vi "lab1_usrp_byte_packet_transceiver.vi"() -> ()   [LabVIEW 2014]
uses:
  <vilib>/addons/Modulation/Analog/support/mod_Set Error Source.vi
  sub_var_stop.vi
  <vilib>/addons/Modulation/Digital/General/MT Generate PSK System Parameters(M).vi
  <vilib>/addons/Modulation/Digital/Support/Common/Validators/mod_Generate Filter Coefficients Validate.vi
  <vilib>/addons/Modulation/Digital/General/subVIs/mod_Generate Filter Coefficients.vi
  <vilib>/addons/Modulation/Digital/General/MT Apply Matched Filter (Generic).vi
  <vilib>/addons/Modulation/Digital/General/MT Align to Ideal Symbols (Generic).vi
  <vilib>/addons/Modulation/Digital/General/MT Map PSK Symbols to Bits.vi
  <instrlib>/niUSRP/niUSRP Fetch Rx Data (CDB Cluster).vi
  <instrlib>/niUSRP/niUSRP Write Tx Data (CDB Cluster).vi
  <vilib>/addons/Modulation/Digital/General/MT Map Bits to PSK Symbols.vi
  <vilib>/addons/Modulation/Digital/General/MT Apply Pulse Shaping Filter (Generic).vi
  <vilib>/addons/Modulation/niDMT.lvlib
panel:
  out "Received symbols":cdb[](graph)
  in  "Transmit power (db)":dbl
  out "History":string
  out "Constellation Map":cdb[](graph)
  out "Received texts":string
  out "Instant rx texts":string
  in  "Instant transmit message":string
  out "size(s) 4":i32
  in  "Send":bool
  out "# elements in buffer":i32
  in  "filter length (symbols)":i32=8
  in  "filter parameter":dbl=0.35 format="%.2f"
  in  "pulse shaping filter (none)":T1(ring)=enum."Raised Cosine"
  in  "M-PSK (4)":i32=4
  in  "samples per symbol (16)":i32=4
  in  "number of samples":i64=40000
  out "coerced gain 2":dbl format="%#_6f"
  out "coerced carrier frequency 2":dbl=915000000.0 format="%#_6p"
  out "coerced IQ rate 2":dbl=4000000.0 format="%#_6p"
  in  "active antenna 2":string="RX2"
  in  "gain 2":dbl format="%#_6f"
  in  "RX device names":refnum<k15>="192.168.10.2"
  out "coerced gain":dbl format="%#_6f"
  out "coerced carrier frequency":dbl=915000000.0 format="%#_6p"
  out "coerced IQ rate":dbl=4000000.0 format="%#_6p"
  in  "TX device names":refnum<k15>="192.168.10.2"
  in  "gain":dbl format="%#_6f"
  in  "carrier frequency":dbl=915000000.0 format="%#_6p"
  in  "IQ rate":dbl=1000000.0 format="%#_6p"
  in  "active antenna":string="TX1"
  in  "stop":bool
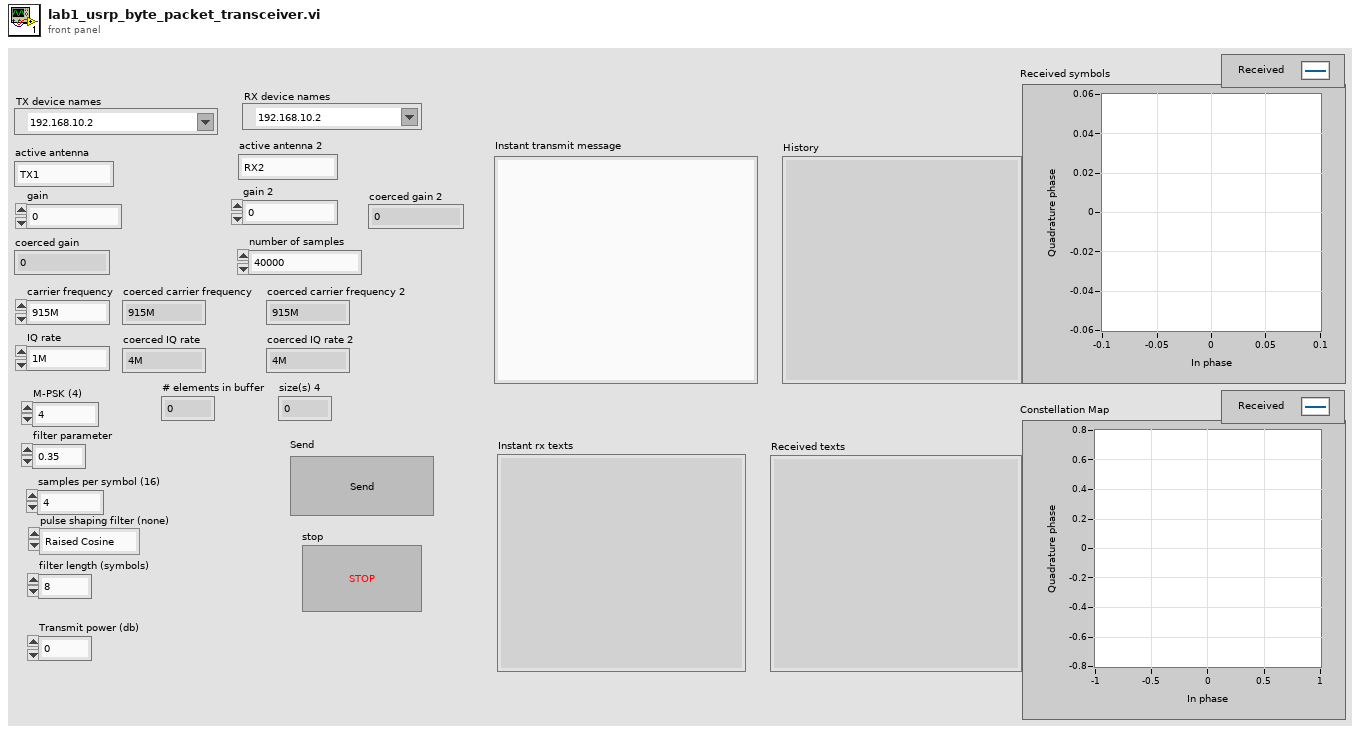
[diagram p1: front panel]
types:
  T1 = enum16{"none", "Raised Cosine", "Root Raised Cos", "Gaussian"}
  T2 = enum16{"FSK", "PSK", "QAM", "MSK", "PAM", "ASK", "CPM"}
  T3 = cluster{"samples per symbol (16)":i32, "symbol map":cdb[], "differential PSK":enum16{"disable", "enable"}, "PSK type":u16}
  T4 = typedef "niAMT.lvlib/Complex Data Waveform.ctl" = cluster{"t0":dbl, "dt":dbl, "Y":cdb[]}
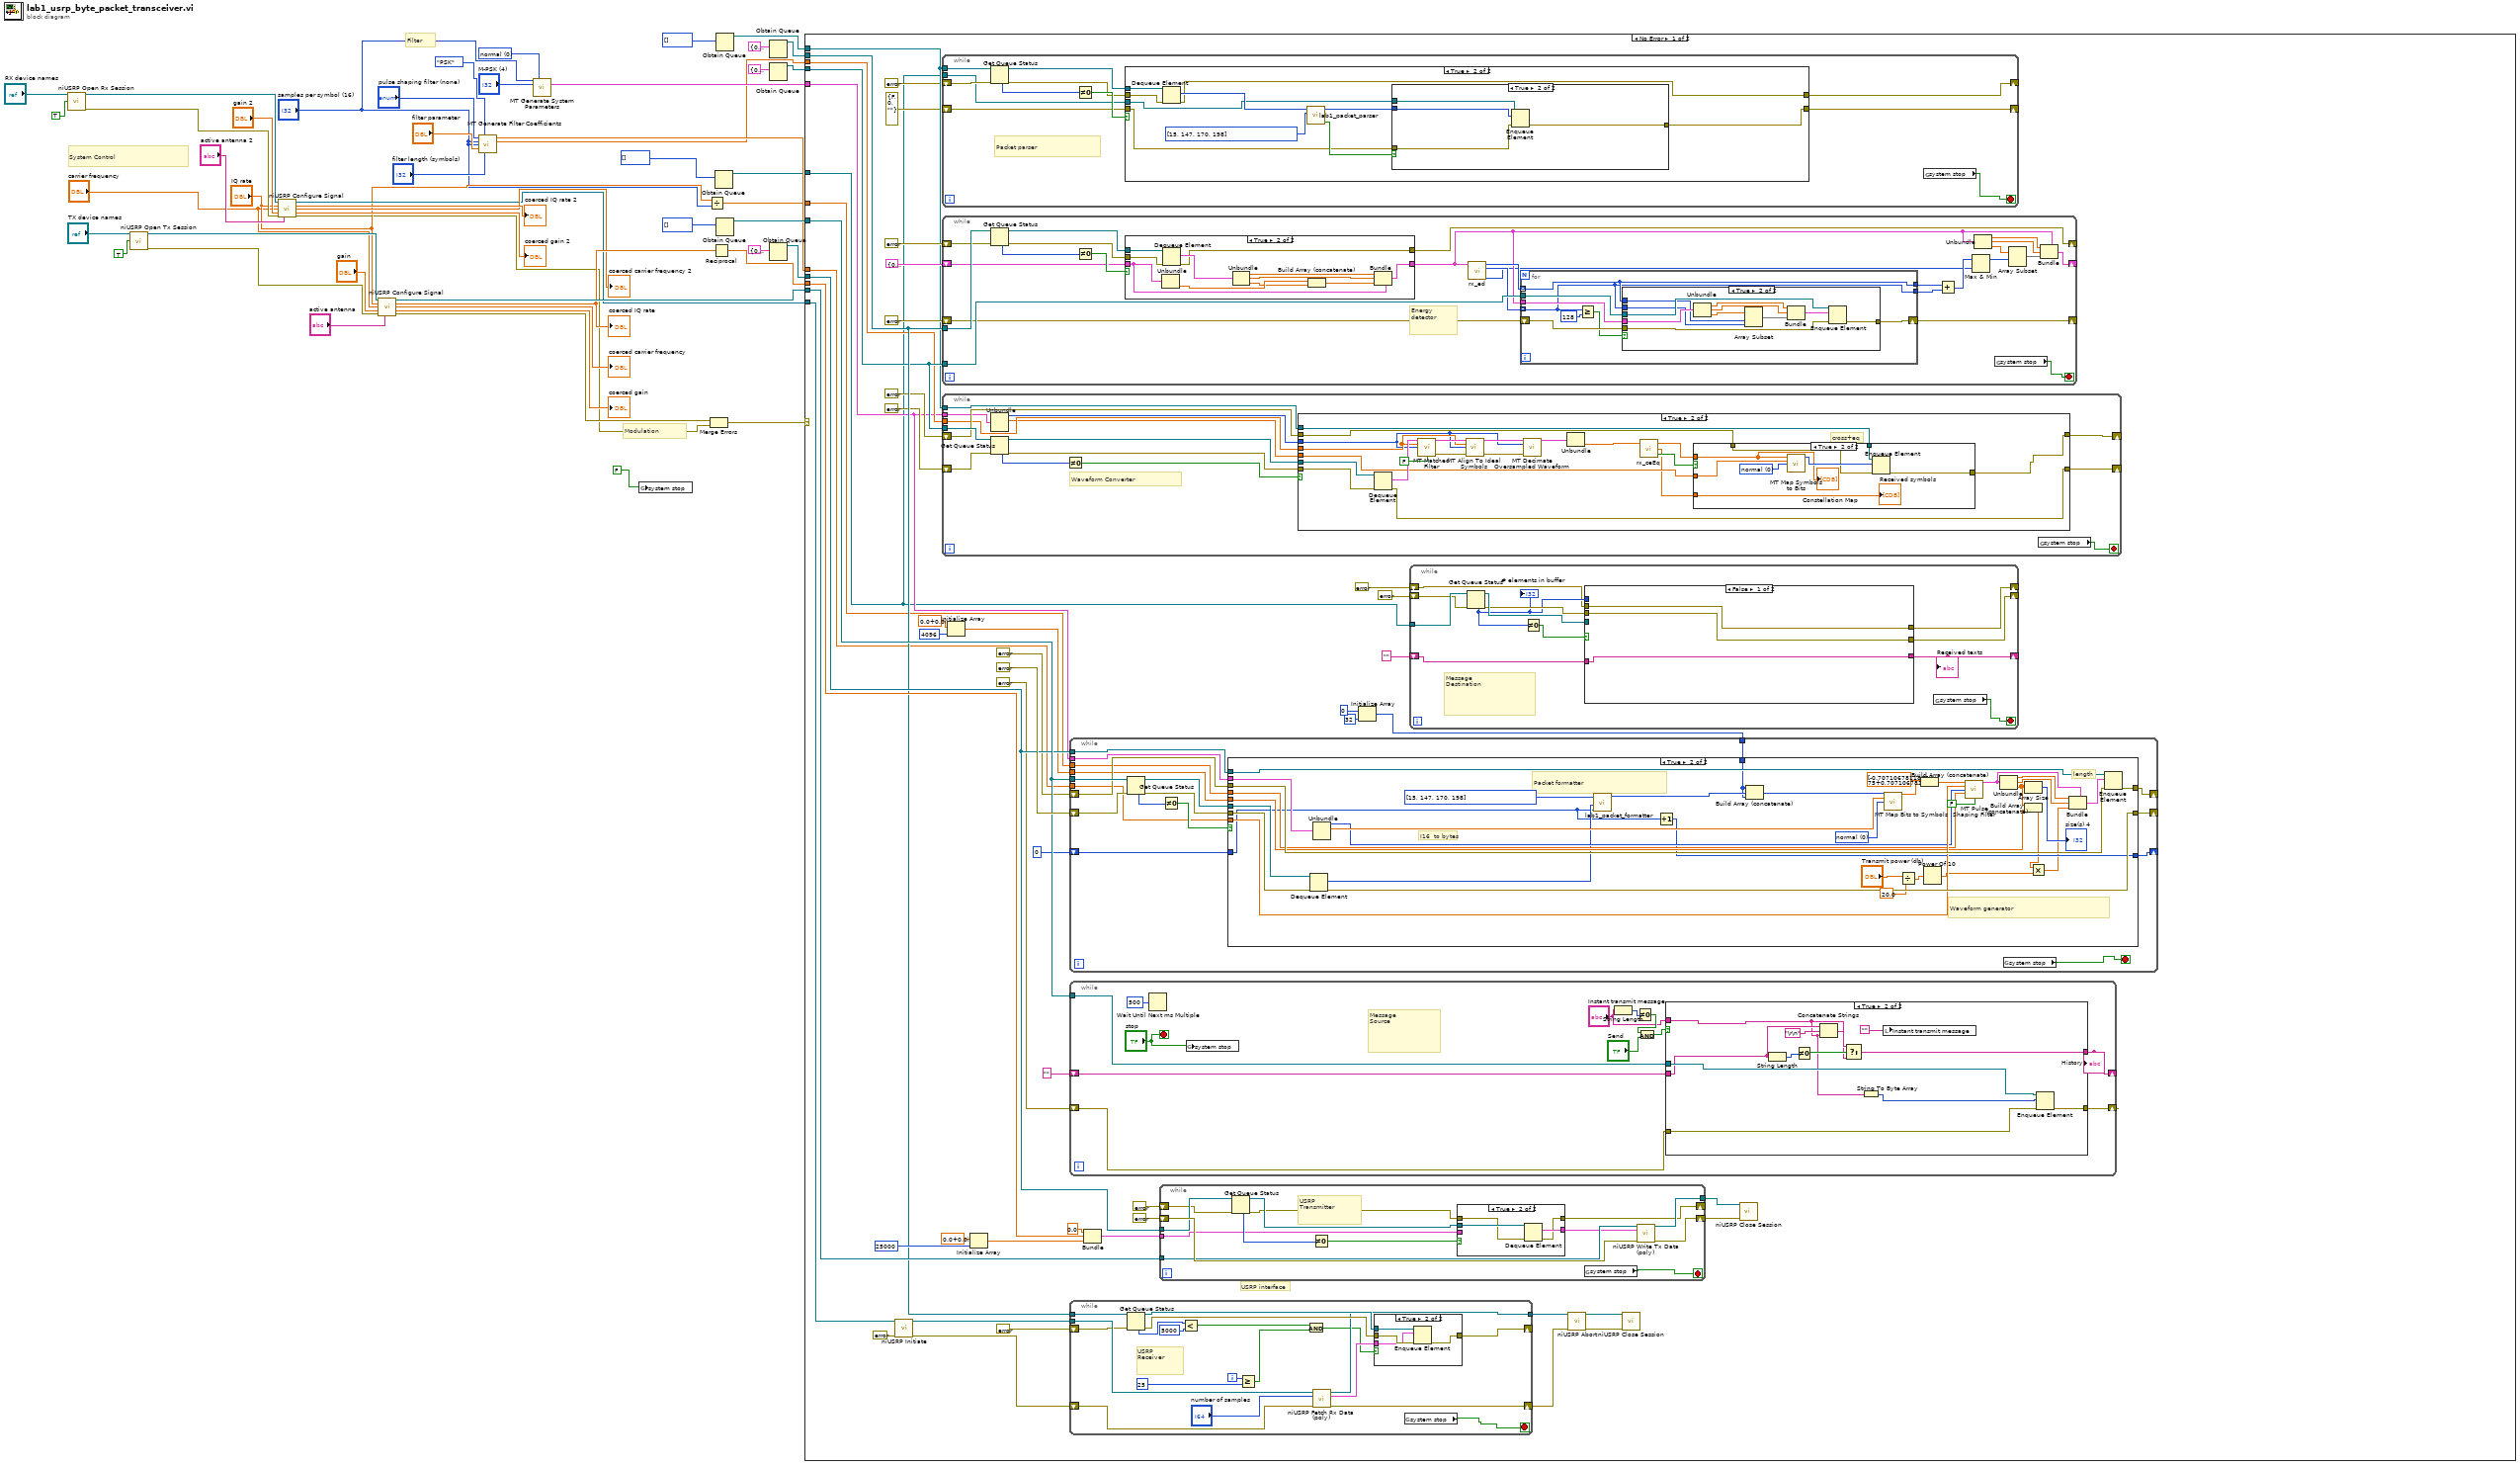
[diagram p0: block diagram]
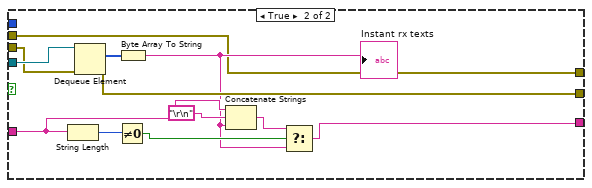
[diagram p2: hidden frame]
diagram:
  w19 = u16 0 items=["normal", "shifted", "offset"] ("PSK type")
  # "Modulation"
  # "Filter"
  # "System Control"
  n1 = call <instrlib>:"niUSRP Open Rx Session.vi"("device names"="RX device names", "reset"=TRUE) -> ("session handle out"=w36:refnum<k15>, "error out"=w35:errorcluster)  [unwired: 12 in]
  n2 = call <instrlib>:"niUSRP Open Tx Session.vi"("device names"="TX device names", "reset"=TRUE) -> ("session handle out"=w49:refnum<k15>, "error out"=w48:errorcluster)  [unwired: 12 in]
  n3 = call <instrlib>:"niUSRP Configure Signal.vi"("session handle"=w36, "IQ rate"="IQ rate", "carrier frequency"="carrier frequency", "gain"="gain 2", "error in (no error)"=w35, "active antenna"="active antenna 2") -> ("session handle out"=w27:refnum<k15>, "coerced IQ rate"=→"coerced IQ rate 2":dbl, "coerced carrier frequency"=→"coerced carrier frequency 2":dbl, "coerced gain"=→"coerced gain 2":dbl, "error out"=w7:errorcluster)  [unwired: 5 in]
  n4 = call <instrlib>:"niUSRP Configure Signal.vi"("session handle"=w49, "IQ rate"="IQ rate", "carrier frequency"="carrier frequency", "gain"="gain", "error in (no error)"=w48, "active antenna"="active antenna") -> ("session handle out"=w40:refnum<k15>, "coerced IQ rate"=w38:dbl, "coerced carrier frequency"=→"coerced carrier frequency":dbl, "coerced gain"=→"coerced gain":dbl, "error out"=w8:errorcluster)  [unwired: 5 in]
  "coerced IQ rate" <- w38
  n5 = call <vilib>:"MT Generate Filter Coefficients.vi"("pulse shaping filter (none)"="pulse shaping filter (none)", "modulation type"=T2."PSK", "pulse shaping samples per symbol (16)"="samples per symbol (16)", "matched samples per symbol (16)"="samples per symbol (16)", "filter parameter"="filter parameter", "filter length (symbols)"="filter length (symbols)") -> ("pulse shaping filter coefficients"=w13:dbl[], "matched filter coefficients"=w11:dbl[])  [unwired: 7 in, 1 out]
  n6 = call-poly <vilib>:"MT Generate System Parameters.vi"("samples per symbol (16)"="samples per symbol (16)", "PSK type"=w19, "M-PSK (4)"="M-PSK (4)") -> ("PSK system parameters"=w14:T3)  [unwired: 10 in, 2 out]
  n7 = global write "sub_var_stop.vi" "system stop"(FALSE) -> ()
  n8 = Divide(x="IQ rate", y="samples per symbol (16)") -> (x/y=w12:dbl)
  n9 = Merge Errors(w8, w7) -> (w6:errorcluster)
  n10 = Reciprocal(x=w38) -> (1/x=w37:dbl)
  n11 = Obtain Queue(element data type=u8[] [] ("payload bytes")) -> (queue out=w4:refnum<queue>)  [unwired: 4 in, 2 out]
  n12 = Obtain Queue(element data type=i8[] [] ("output bit stream")) -> (queue out=w22:refnum<queue>)  [unwired: 4 in, 2 out]
  n13 = Obtain Queue(element data type=i16[] []) -> (queue out=w50:refnum<queue>)  [unwired: 4 in, 2 out]
  n14 = Obtain Queue(element data type=cluster{"t0":dbl, "dt":dbl, "Y":cdb[]} {"t0"=0.0, "dt"=0.0, "Y"=[]} ("data")) -> (queue out=w26:refnum<queue>)  [unwired: 4 in, 2 out]
  n15 = Obtain Queue(element data type=cluster{"t0":dbl, "dt":dbl, "Y":cdb[]} {"t0"=0.0, "dt"=0.0, "Y"=[]} ("data")) -> (queue out=w23:refnum<queue>)  [unwired: 4 in, 2 out]
  n16 = Obtain Queue(element data type=cluster{"t0":dbl, "dt":dbl, "Y":cdb[]} {"t0"=0.0, "dt"=1.0, "Y"=[]} ("data")) -> (queue out=w41:refnum<queue>)  [unwired: 4 in, 2 out]
  n17 = case shown="No Error" w6 {
    tunnel: w50 -> [w100 _]
    tunnel: w41 -> [w95 _]
    tunnel: w40 -> [w96 _]
    tunnel: w37 -> [w89 _]
    tunnel: w27 -> [w84 _]
    tunnel: w26 -> [w78 _]
    tunnel: w23 -> [w74 _]
    tunnel: w22 -> [w72 _]
    tunnel: w14 -> [w66 _]
    tunnel: w13 -> [w69 _]
    tunnel: w12 -> [w68 _]
    tunnel: w11 -> [w67 _]
    tunnel: w4 -> [w59 _]
    frame No Error {
      # "USRP interface"
      n18 = call <instrlib>:"niUSRP Initiate.vi"("session handle"=w84, "error in (no error)"=errorcluster {"status"=FALSE, "code"=0, "source"=""}) -> ("session handle out"=w83:refnum<k15>, "error out"=w82:errorcluster)  [unwired: 12 in]
      n19 = while {
        tunnel: w72 -> [w139]
        shift-right: [w130] -> _
        shift-left: errorcluster {"status"=FALSE, "code"=0, "source"=""} ("error out") -> [w138]
        tunnel: w59 -> [w133]
        shift-right: [w132] -> _
        shift-left: errorcluster {"status"=FALSE, "code"=0, "source"=""} ("error out") -> [w131]
        stop <- w129 stop-if-true
        # "Packet parser"
        n20 = Get Queue Status(queue=w139, error in (no error)=w138) -> (queue out=w135:refnum<queue>, error out=w134:errorcluster, # elements in queue=w137:i32)  [unwired: 1 in, 5 out]
        n21 = Not Equal To 0?(x=w137) -> (x != 0?=w136:bool)
        n22 = case shown="True" w136 {
          tunnel: w135 -> [_ w151]
          tunnel: w134 -> [w140 w150]
          tunnel: w133 -> [_ w144]
          tunnel: [w141 w142] -> w132
          tunnel: w131 -> [w141 w143]
          tunnel: [w140 w145] -> w130
          frame False {
          }
          frame True {
            n23 = Dequeue Element(queue=w151, error in (no error)=w150) -> (element=w149:i8[], error out=w145:errorcluster)  [unwired: 1 in, 2 out]
            n24 = call "lab1_packet_parser.vi"("preamble bytes"=u8[] [15, 147, 170, 198] ("Array"), "bitstream"=w149) -> ("Found?"=w147:bool, "payload bytes"=w146:u8[])  [unwired: 6 in, 2 out]
            n25 = case shown="True" w147 {
              tunnel: w146 -> [_ w156]
              tunnel: w144 -> [_ w155]
              tunnel: w143 -> [w152 w154]
              tunnel: [w152 w153] -> w142
              frame False {
              }
              frame True {
                n26 = Enqueue Element(queue=w155, element=w156, error in (no error)=w154) -> (error out=w153:errorcluster)  [unwired: 1 in, 2 out]
              }
            }
          }
        }
        n27 = global read "sub_var_stop.vi" "system stop"() -> (w129:bool)
      }
      n28 = while {
        tunnel: w78 -> [w227]
        shift-right: [w220] -> _
        shift-left: errorcluster {"status"=FALSE, "code"=0, "source"=""} ("error out") -> [w226]
        shift-right: [w207] -> _
        shift-left: cluster{"t0":dbl, "dt":dbl, "Y":cdb[]} {"t0"=0.0, "dt"=0.0, "Y"=[]} ("data") -> [w221]
        tunnel: w74 -> [w219]
        shift-right: [w218] -> _
        shift-left: errorcluster {"status"=FALSE, "code"=0, "source"=""} ("error out") -> [w217]
        stop <- w203 stop-if-true
        # "Energy\ndetector"
        n29 = Get Queue Status(queue=w227, error in (no error)=w226) -> (queue out=w222:refnum<queue>, error out=w223:errorcluster, # elements in queue=w225:i32)  [unwired: 1 in, 5 out]
        n30 = Not Equal To 0?(x=w225) -> (x != 0?=w224:bool)
        n31 = case shown="True" w224 {
          tunnel: w223 -> [w249 w260]
          tunnel: w222 -> [_ w259]
          tunnel: w221 -> [w248 w254]
          tunnel: [w249 w251] -> w220
          tunnel: [w248 w250] -> w214
          frame False {
          }
          frame True {
            n32 = Unbundle(w254) -> ("Y"=w257:cdb[])  [unwired: 2 out]
            n33 = Dequeue Element(queue=w259, error in (no error)=w260) -> (element=w258:cluster{"t0":dbl, "dt":dbl, "Y":cdb[]}, error out=w251:errorcluster)  [unwired: 1 in, 2 out]
            n34 = Unbundle(w258) -> ("t0"=w253:dbl, "dt"=w252:dbl, "Y"=w256:cdb[])
            n35 = Build Array (concatenate)(w257, w256) -> (w255:cdb[])
            n36 = Bundle(cluster=w254, "t0"=w253, "dt"=w252, "Y"=w255) -> (w250:cluster{"t0":dbl, "dt":dbl, "Y":cdb[]})
          }
        }
        n37 = call "rx_ed.vi"("Wavefrom"=w214) -> ("first pulse"=w204:i32, "length"=w215:i32[], "start index"=w216:i32[])  [unwired: 7 in, 1 out]
        n38 = for {
          tunnel: w219 -> [w235]
          tunnel: w214 -> [w232]
          shift-right: [w234] -> w218
          shift-left: w217 -> [w233]
          tunnel: w216 -> [w231] mode=indexing
          tunnel: w215 -> [w230] mode=indexing
          tunnel: [w231] -> w210
          tunnel: [w230] -> w209
          n39 = Greater Or Equal?(x=w230, y=128) -> (x >= y?=w228:bool)
          n40 = case shown="True" w228 {
            tunnel: w235 -> [_ w247]
            tunnel: [w236 w246] -> w234
            tunnel: w233 -> [w236 w245]
            tunnel: w232 -> [_ w244]
            tunnel: w231 -> [_ w238]
            tunnel: w230 -> [_ w237]
            frame False {
            }
            frame True {
              n41 = Unbundle(w244) -> ("t0"=w242:dbl, "dt"=w243:dbl, "Y"=w240:cdb[])
              n42 = Array Subset(array=w240, index=w238, length=w237) -> (w239:cdb[])
              n43 = Bundle("t0"=w242, "dt"=w243, w239) -> (w241:cluster{"t0":dbl, "dt":dbl, cdb[]})  [unwired: 1 in]
              n44 = Enqueue Element(queue=w247, element=w241, error in (no error)=w245) -> (error out=w246:errorcluster)  [unwired: 1 in, 2 out]
            }
          }
        }
        n45 = Add(x=w210, y=w209) -> (x+y=w206:i32)
        n46 = Max & Min(x=w206, y=w204) -> (max(x,y)=w205:i32)  [unwired: 1 out]
        n47 = Unbundle(w214) -> ("t0"=w213:dbl, "dt"=w212:dbl, "Y"=w211:cdb[])
        n48 = global read "sub_var_stop.vi" "system stop"() -> (w203:bool)
        n49 = Array Subset(array=w211, index=w205) -> (w208:cdb[])  [unwired: 1 in]
        n50 = Bundle(cluster=w214, "t0"=w213, "dt"=w212, "Y"=w208) -> (w207:cluster{"t0":dbl, "dt":dbl, "Y":cdb[]})
      }
      n51 = while {
        tunnel: w74 -> [w171]
        shift-right: [w165] -> _
        shift-left: errorcluster {"status"=FALSE, "code"=0, "source"=""} ("error out") -> [w170]
        tunnel: w72 -> [w164]
        shift-right: [w163] -> _
        shift-left: errorcluster {"status"=FALSE, "code"=0, "source"=""} ("error out") -> [w162]
        tunnel: w67 -> [w161]
        tunnel: w66 -> [w160]
        stop <- w157 stop-if-true
        # "Waveform Converter"
        n52 = Unbundle(w160) -> ("samples per symbol (16)"=w159:i32, "symbol map"=w158:cdb[])  [unwired: 2 out]
        n53 = Get Queue Status(queue=w171, error in (no error)=w170) -> (queue out=w167:refnum<queue>, error out=w166:errorcluster, # elements in queue=w169:i32)  [unwired: 1 in, 5 out]
        n54 = Not Equal To 0?(x=w169) -> (x != 0?=w168:bool)
        n55 = case shown="True" w168 {
          tunnel: w167 -> [_ w192]
          tunnel: w166 -> [w173 w193]
          tunnel: [w173 w191] -> w165
          tunnel: w164 -> [_ w177]
          tunnel: [w172 w175] -> w163
          tunnel: w162 -> [w172 w176]
          tunnel: w161 -> [_ w183]
          tunnel: w159 -> [_ w182]
          tunnel: w158 -> [_ w181]
          frame False {
          }
          frame True {
            # "cross+eq"
            n56 = Dequeue Element(queue=w192, error in (no error)=w193) -> (element=w190:cluster{"t0":dbl, "dt":dbl, "Y":cdb[]}, error out=w191:errorcluster)  [unwired: 1 in, 2 out]
            n57 = call-poly <vilib>:"MT Matched Filter.vi"("input complex waveform"=w190, "matched filter coefficients"=w183, "samples per symbol (16)"=w182, "reset? (T)"=FALSE) -> ("output complex waveform"=w189:T4, "error out"=w188:errorcluster)  [unwired: 10 in]
            n58 = call-poly <vilib>:"MT Align To Ideal Symbols.vi"("input complex waveform"=w189, "matched filter coefficients"=w183, "samples per symbol (16)"=w182, "error in (no error)"=w188) -> ("output complex waveform"=w186:T4, "error out"=w187:errorcluster)  [unwired: 9 in, 1 out]
            n59 = call <vilib>:"MT Decimate Oversampled Waveform.vi"("input complex waveform"=w186, "decimation factor"=w182, "error in (no error)"=w187) -> ("output complex waveform"=w185:T4)  [unwired: 11 in, 1 out]
            n60 = Unbundle(w185) -> ("Y"=w184:cdb[])  [unwired: 2 out]
            n61 = call "rx_ceEq.vi"("symbols"=w184) -> ("valid?"=w179:bool, "neq symbols"=w174:cdb[], "eq symbols"=w180:cdb[])  [unwired: 2 in]
            n62 = case shown="True" w179 {
              tunnel: w181 -> [_ w202]
              tunnel: w180 -> [_ w196]
              tunnel: w177 -> [_ w199]
              tunnel: w176 -> [w194 w198]
              tunnel: [w194 w197] -> w175
              tunnel: w174 -> [_ w195]
              frame False {
              }
              frame True {
                w201 = u16 0 items=["normal", "shifted", "offset"] ("PSK type")
                n63 = call-poly <vilib>:"MT Map Symbols to Bits.vi"("symbols"=w196, "symbol map"=w202, "PSK type"=w201) -> ("output bit stream"=w200:i8[])  [unwired: 11 in, 1 out]
                n64 = Enqueue Element(queue=w199, element=w200, error in (no error)=w198) -> (error out=w197:errorcluster)  [unwired: 1 in, 2 out]
                "Constellation Map" <- w196
                "Received symbols" <- w195
              }
            }
          }
        }
        n65 = global read "sub_var_stop.vi" "system stop"() -> (w157:bool)
      }
      n66 = Initialize Array(cdb 0.0+0.0i, 4096) -> (w61:cdb[])
      n67 = Initialize Array(cdb 0.0+0.0i, 25000 ("dimension size")) -> (w90:cdb[])
      n68 = while {
        tunnel: w100 -> [w372]
        shift-right: [w370] -> _
        shift-left: errorcluster {"status"=FALSE, "code"=0, "source"=""} ("error out") -> [w371]
        shift-right: [w363] -> _
        shift-left: "" -> [w369]
        stop <- "stop" stop-if-true
        # "Message\nSource"
        n69 = Wait Until Next ms Multiple(millisecond multiple=u32 500) -> ()  [unwired: 1 out]
        n70 = global write "sub_var_stop.vi" "system stop"("stop") -> ()
        n71 = String Length(string="Instant transmit message") -> (length=w368:i32)
        n72 = Not Equal To 0?(x=w368) -> (x != 0?=w367:bool)
        n73 = And(x=w367, y="Send") -> (x .and. y?=w365:bool)
        n74 = case shown="True" w365 {
          tunnel: w372 -> [_ w387]
          tunnel: w371 -> [w375 w386]
          tunnel: [w375 w385] -> w370
          tunnel: w369 -> [w374 w381]
          tunnel: "Instant transmit message" -> [_ w378]
          tunnel: [w374 w379] -> w363
          frame False {
          }
          frame True {
            n75 = String Length(string=w381) -> (length=w384:i32)
            n76 = Not Equal To 0?(x=w384) -> (x != 0?=w383:bool)
            n77 = Concatenate Strings(w381, "\r\n", w378) -> (w380:string)
            n78 = Select(t=w380, s=w383, f=w378) -> (s? t:f=w379:string)
            n79 = String To Byte Array(string=w378) -> (unsigned byte array=w377:u8[])
            n80 = local write "Instant transmit message"("") -> ()
            n81 = Enqueue Element(queue=w387, element=w377, error in (no error)=w386) -> (error out=w385:errorcluster)  [unwired: 1 in, 2 out]
          }
        }
        "History" <- w363
      }
      n82 = while {
        tunnel: w83 -> [w279]
        shift-right: [w267] -> w79
        shift-left: w82 -> [w278]
        tunnel: w78 -> [w276]
        shift-right: [w270] -> _
        shift-left: errorcluster {"status"=FALSE, "code"=0, "source"=""} ("error out") -> [w275]
        tunnel: [w268] -> w80
        i -> [w266]
        stop <- w261 stop-if-true
        # "USRP\nReceiver"
        n83 = Get Queue Status(queue=w276, error in (no error)=w275) -> (queue out=w272:refnum<queue>, error out=w271:errorcluster, # elements in queue=w274:i32)  [unwired: 1 in, 5 out]
        n84 = Less?(x=w274, y=5000) -> (x < y?=w264:bool)
        n85 = Greater Or Equal?(x=w266, y=25) -> (x >= y?=w263:bool)
        n86 = And(x=w264, y=w263) -> (x .and. y?=w262:bool)
        n87 = call-poly <instrlib>:"niUSRP Fetch Rx Data (poly).vi"("session handle"=w279, "number of samples"="number of samples", "error in (no error)"=w278) -> ("session handle out"=w268:refnum<k15>, "data"=w269:cluster{"t0":dbl, "dt":dbl, "Y":cdb[]}, "error out"=w267:errorcluster)  [unwired: 9 in, 1 out]
        n88 = case shown="True" w262 {
          tunnel: w272 -> [_ w284]
          tunnel: w271 -> [w280 w283]
          tunnel: [w280 w282] -> w270
          tunnel: w269 -> [_ w281]
          frame False {
          }
          frame True {
            n89 = Enqueue Element(queue=w284, element=w281, error in (no error)=w283) -> (error out=w282:errorcluster)  [unwired: 1 in, 2 out]
          }
        }
        n90 = global read "sub_var_stop.vi" "system stop"() -> (w261:bool)
      }
      n91 = Bundle(0.0, w89, w90) -> (w87:cluster{dbl, dbl, cdb[]})  [unwired: 1 in]
      n92 = while {
        shift-right: [w294] -> w99
        shift-left: errorcluster {"status"=FALSE, "code"=0, "source"=""} ("error out") -> [w292]
        tunnel: [w293] -> w98
        tunnel: w96 -> [w291]
        tunnel: w95 -> [w289]
        shift-right: [w287] -> _
        shift-left: errorcluster {"status"=FALSE, "code"=0, "source"=""} ("error out") -> [w288]
        tunnel: w87 -> [w286]
        stop <- w285 stop-if-true
        # "USRP\nTransmitter"
        n93 = Get Queue Status(queue=w289, error in (no error)=w288) -> (queue out=w296:refnum<queue>, error out=w295:errorcluster, # elements in queue=w298:i32)  [unwired: 1 in, 5 out]
        n94 = Not Equal To 0?(x=w298) -> (x != 0?=w297:bool)
        n95 = case shown="True" w297 {
          tunnel: w296 -> [_ w304]
          tunnel: w295 -> [w299 w303]
          tunnel: [w300 w302] -> w290
          tunnel: [w299 w301] -> w287
          tunnel: w286 -> [w300 _]
          frame False {
          }
          frame True {
            n96 = Dequeue Element(queue=w304, error in (no error)=w303) -> (element=w302:cluster{"t0":dbl, "dt":dbl, "Y":cdb[]}, error out=w301:errorcluster)  [unwired: 1 in, 2 out]
          }
        }
        n97 = global read "sub_var_stop.vi" "system stop"() -> (w285:bool)
        n98 = call-poly <instrlib>:"niUSRP Write Tx Data (poly).vi"("session handle"=w291, "data"=w290, "error in (no error)"=w292) -> ("session handle out"=w293:refnum<k15>, "error out"=w294:errorcluster)  [unwired: 11 in]
      }
      n99 = Initialize Array(0, 32 ("dimension size")) -> (w51:i32[])
      n100 = while {
        tunnel: w100 -> [w319]
        shift-right: [w316] -> _
        shift-left: errorcluster {"status"=FALSE, "code"=0, "source"=""} ("error out") -> [w322]
        tunnel: w95 -> [w315]
        shift-right: [w314] -> _
        shift-left: errorcluster {"status"=FALSE, "code"=0, "source"=""} ("error out") -> [w313]
        tunnel: w66 -> [w312]
        tunnel: w69 -> [w311]
        tunnel: w68 -> [w310]
        tunnel: w61 -> [w309]
        shift-right: [w307] -> _
        shift-left: 0 -> [w308]
        tunnel: w51 -> [w306]
        stop <- w305 stop-if-true
        n101 = Get Queue Status(queue=w319, error in (no error)=w322) -> (queue out=w317:refnum<queue>, error out=w318:errorcluster, # elements in queue=w321:i32)  [unwired: 1 in, 5 out]
        n102 = Not Equal To 0?(x=w321) -> (x != 0?=w320:bool)
        n103 = case shown="True" w320 {
          tunnel: w318 -> [w325 w361]
          tunnel: w317 -> [_ w360]
          tunnel: [w325 w359] -> w316
          tunnel: w315 -> [_ w358]
          tunnel: [w324 w357] -> w314
          tunnel: w313 -> [w324 w356]
          tunnel: w312 -> [_ w352]
          tunnel: w311 -> [_ w351]
          tunnel: w310 -> [_ w350]
          tunnel: w309 -> [_ w346]
          tunnel: w308 -> [w323 w337]
          tunnel: [w323 w336] -> w307
          tunnel: w306 -> [_ w333]
          frame False {
          }
          frame True {
            w347 = u16 0 items=["normal", "shifted", "offset"] ("PSK type")
            # "Waveform generator"
            # "length"
            # "I16  to bytes"
            # "Packet formatter"
            n104 = Dequeue Element(queue=w360, error in (no error)=w361) -> (element=w338:i16[], error out=w359:errorcluster)  [unwired: 1 in, 2 out]
            n105 = Unbundle(w352) -> ("samples per symbol (16)"=w348:i32, "symbol map"=w349:cdb[])  [unwired: 2 out]
            n106 = call "lab1_packet_formatter.vi"("counter"=w337, "payload(bytes array)"=w338, "preamble(bytes array)"=u8[] [15, 147, 170, 198] ("Array")) -> ("bitstream"=w334:i16[])  [unwired: 8 in]
            n107 = Increment(x=w337) -> (x+1=w336:i32)
            n108 = Build Array (concatenate)(w333, w334, w333) -> (w332:i32[])
            n109 = call-poly <vilib>:"MT Map Bits to Symbols.vi"("input bit stream"=w332, "symbol map"=w349, "PSK type"=w347) -> ("symbols"=w354:cdb[])  [unwired: 11 in, 1 out]
            n110 = Divide(x="Transmit power (db)", y=20.0) -> (x/y=w329:dbl)
            n111 = Build Array (concatenate)(cdb[] [-0.7071067811865475+0.7071067811865476i, 0.7071067811865476+0.7071067811865475i, 0.7071067811865474-0.7071067811865477i, 0.7071067811865476+0.7071067811865475i, -0.7071067811865475+0.7071067811865476i, -0.7071067811865477-0.7071067811865475i, 0.7071067811865476+0.7071067811865475i, -0.7071067811865477-0.7071067811865475i, -0.7071067811865475+0.7071067811865476i, 0.7071067811865476+0.7071067811865475i, 0.7071067811865474-0.7071067811865477i, 0.7071067811865476+0.7071067811865475i, -0.7071067811865475+0.7071067811865476i, -0.7071067811865477-0.7071067811865475i, 0.7071067811865476+0.7071067811865475i, -0.7071067811865477-0.7071067811865475i, -0.7071067811865475+0.7071067811865476i, 0.7071067811865476+0.7071067811865475i, 0.7071067811865474-0.7071067811865477i, 0.7071067811865476+0.7071067811865475i, -0.7071067811865475+0.7071067811865476i, -0.7071067811865477-0.7071067811865475i, 0.7071067811865476+0.7071067811865475i, -0.7071067811865477-0.7071067811865475i, -0.7071067811865475+0.7071067811865476i, 0.7071067811865476+0.7071067811865475i, 0.7071067811865474-0.7071067811865477i, 0.7071067811865476+0.7071067811865475i, -0.7071067811865475+0.7071067811865476i, -0.7071067811865477-0.7071067811865475i, 0.7071067811865476+0.7071067811865475i, -0.7071067811865477-0.7071067811865475i, -0.7071067811865475+0.7071067811865476i, 0.7071067811865476+0.7071067811865475i, 0.7071067811865474-0.7071067811865477i, 0.7071067811865476+0.7071067811865475i, -0.7071067811865475+0.7071067811865476i, -0.7071067811865477-0.7071067811865475i, 0.7071067811865476+0.7071067811865475i, -0.7071067811865477-0.7071067811865475i, -0.7071067811865475+0.7071067811865476i, 0.7071067811865476+0.7071067811865475i, 0.7071067811865474-0.7071067811865477i, 0.7071067811865476+0.7071067811865475i, -0.7071067811865475+0.7071067811865476i, -0.7071067811865477-0.7071067811865475i, 0.7071067811865476+0.7071067811865475i, -0.7071067811865477-0.7071067811865475i, -0.7071067811865475+0.7071067811865476i, 0.7071067811865476+0.7071067811865475i, 0.7071067811865474-0.7071067811865477i, 0.7071067811865476+0.7071067811865475i, -0.7071067811865475+0.7071067811865476i, -0.7071067811865477-0.7071067811865475i, 0.7071067811865476+0.7071067811865475i, -0.7071067811865477-0.7071067811865475i, -0.7071067811865475+0.7071067811865476i, 0.7071067811865476+0.7071067811865475i, 0.7071067811865474-0.7071067811865477i, 0.7071067811865476+0.7071067811865475i, -0.7071067811865475+0.7071067811865476i, -0.7071067811865477-0.7071067811865475i, 0.7071067811865476+0.7071067811865475i, -0.7071067811865477-0.7071067811865475i] ("symbols"), w354) -> (w353:cdb[])
            n112 = Power Of 10(x=w329) -> (10^x=w328:dbl)
            n113 = call-poly <vilib>:"MT Pulse Shaping Filter.vi"("symbols"=w353, "pulse shaping filter coefficients"=w351, "samples per symbol (16)"=w348, "symbol rate (Hz)"=w350, "reset? (T)"=FALSE) -> ("output complex waveform"=w345:T4)  [unwired: 9 in, 1 out]
            n114 = Unbundle(w345) -> ("t0"=w344:dbl, "dt"=w343:dbl, "Y"=w341:cdb[])
            n115 = Array Size(array=w341) -> (size(s)=→"size(s) 4":i32)
            n116 = Build Array (concatenate)(w341, w346) -> (w327:cdb[])
            n117 = Multiply(x=w327, y=w328) -> (x*y=w326:cdb[])
            n118 = Bundle(cluster=w345, "t0"=w344, "dt"=w343, "Y"=w326) -> (w342:T4)
            n119 = Enqueue Element(queue=w358, element=w342, error in (no error)=w356) -> (error out=w357:errorcluster)  [unwired: 1 in, 2 out]
          }
        }
        n120 = global read "sub_var_stop.vi" "system stop"() -> (w305:bool)
      }
      n121 = while {
        tunnel: w59 -> [w113]
        shift-right: [w106] -> _
        shift-left: errorcluster {"status"=FALSE, "code"=0, "source"=""} ("error out") -> [w107]
        shift-right: [w109] -> _
        shift-left: errorcluster {"status"=FALSE, "code"=0, "source"=""} ("error out") -> [w110]
        shift-right: [w103] -> _
        shift-left: "" -> [w104]
        stop <- w102 stop-if-true
        # "Message\nDestination"
        n122 = Get Queue Status(queue=w113, error in (no error)=w110) -> (queue out=w112:refnum<queue>, error out=w111:errorcluster, # elements in queue=w108:i32)  [unwired: 1 in, 5 out]
        "# elements in buffer" <- w108
        n123 = Not Equal To 0?(x=w108) -> (x != 0?=w105:bool)
        n124 = case shown="False" w105 {
          tunnel: w112 -> [_ w128]
          tunnel: w111 -> [w116 w127]
          tunnel: [w116 w126] -> w109
          tunnel: w108 -> [_ _]
          tunnel: w107 -> [w115 w117]
          tunnel: [w115 w117] -> w106
          tunnel: w104 -> [w114 w121]
          tunnel: [w114 w118] -> w103
          frame False {
          }
          frame True {
            n125 = String Length(string=w121) -> (length=w124:i32)
            n126 = Dequeue Element(queue=w128, error in (no error)=w127) -> (element=w125:u8[], error out=w126:errorcluster)  [unwired: 1 in, 2 out]
            n127 = Not Equal To 0?(x=w124) -> (x != 0?=w123:bool)
            n128 = Byte Array To String(unsigned byte array=w125) -> (string=w120:string)
            "Instant rx texts" <- w120
            n129 = Concatenate Strings(w121, "\r\n", w120) -> (w119:string)
            n130 = Select(t=w119, s=w123, f=w120) -> (s? t:f=w118:string)
          }
        }
        "Received texts" <- w103
        n131 = global read "sub_var_stop.vi" "system stop"() -> (w102:bool)
      }
      n132 = call <instrlib>:"niUSRP Abort.vi"("session handle"=w80, "error in (no error)"=w79) -> ("session handle out"=w86:refnum<k15>, "error out"=w85:errorcluster)  [unwired: 12 in]
      n133 = call <instrlib>:"niUSRP Close Session.vi"("session handle"=w86, "error in (no error)"=w85) -> ()  [unwired: 13 in, 1 out]
      n134 = call <instrlib>:"niUSRP Close Session.vi"("session handle"=w98, "error in (no error)"=w99) -> ()  [unwired: 13 in, 1 out]
    }
    frame Error {
    }
  }
